vi "EXCOM-TCP-28.vi"(0 "connection ID":refnum<k5>, 5 "Error IN":errorcluster) -> (14 "CID Out":refnum<k5>, 15 "NORA":dbl format="%<%H:%M:%S%0u>t", 16 "NODEC":dbl format="%<%H:%M:%S%0u>t", 17 "DEC":dbl format="%.2f", 18 "HA":dbl format="%.2f", 19 "Error Out":errorcluster)   [LabVIEW 2011]
panel:
  out "Q String":string
  out "RA":dbl format="%<%H:%M:%S%0u>t"
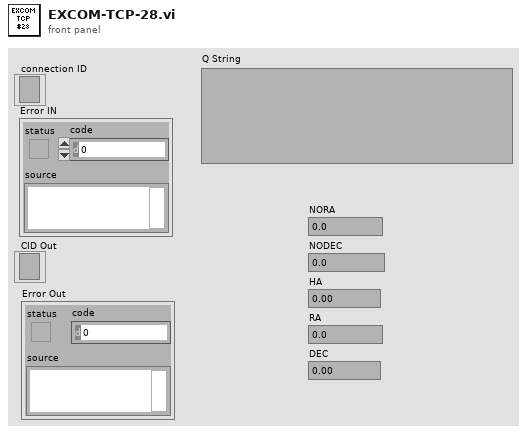
[diagram p1: front panel]
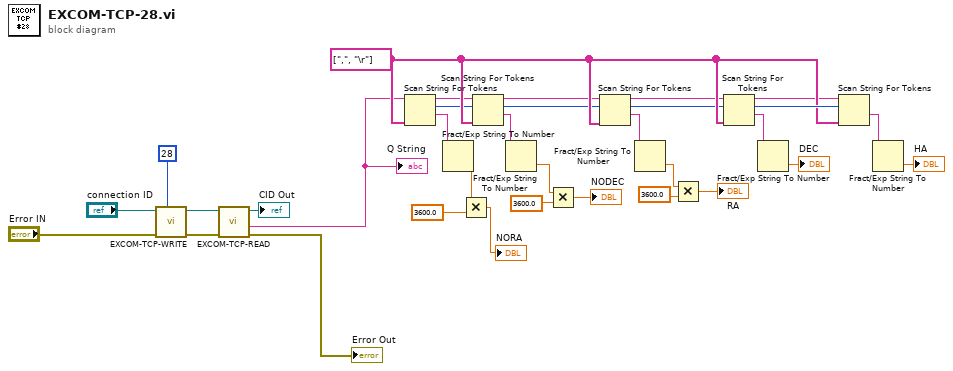
[diagram p0: block diagram]
diagram:
  w25 = string[] [",", "\r"] ("delimiters (\\s,\\t,\\r,\\n)")
  n1 = call "EXCOM-TCP-WRITE.vi"("Commande #"=28, "Error IN"="Error IN", "connection ID"="connection ID") -> ("Error OUT"=w31:errorcluster, "connection ID out"=w30:refnum<k5>)  [unwired: 4 in, 2 out]
  n2 = call "EXCOM-TCP-READ.vi"("Error In"=w31, "connection ID"=w30) -> ("Error Out"=→"Error Out":errorcluster, "Response"=w1:string, "CID Out"=→"CID Out":refnum<k5>)  [unwired: 5 in]
  "Q String" <- w1
  n3 = Scan String For Tokens(6:w25, 9:w1) -> (1:w8:string, 2:w7:i32, 3:w6:string)  [unwired: 4 in, 1 out]
  n4 = Fract/Exp String To Number(string=w8) -> (number=w9:dbl)  [unwired: 3 in, 1 out]
  n5 = Multiply(x=w9, y=3600.0) -> (x*y=→"NORA":dbl)
  n6 = Scan String For Tokens(6:w25, 8:w7, 9:w6) -> (1:w20:string, 2:w4:i32, 3:w5:string)  [unwired: 3 in, 1 out]
  n7 = Fract/Exp String To Number(string=w20) -> (number=w16:dbl)  [unwired: 3 in, 1 out]
  n8 = Multiply(x=w16, y=3600.0) -> (x*y=→"NODEC":dbl)
  n9 = Scan String For Tokens(6:w25, 8:w4, 9:w5) -> (1:w14:string, 2:w2:i32, 3:w3:string)  [unwired: 3 in, 1 out]
  n10 = Fract/Exp String To Number(string=w14) -> (number=w18:dbl)  [unwired: 3 in, 1 out]
  n11 = Multiply(x=w18, y=3600.0) -> (x*y=→"RA":dbl)
  n12 = Scan String For Tokens(6:w25, 8:w2, 9:w3) -> (1:w15:string, 2:w26:i32, 3:w24:string)  [unwired: 3 in, 1 out]
  n13 = Fract/Exp String To Number(string=w15) -> (number=→"DEC":dbl)  [unwired: 3 in, 1 out]
  n14 = Scan String For Tokens(6:w25, 8:w26, 9:w24) -> (1:w23:string)  [unwired: 3 in, 3 out]
  n15 = Fract/Exp String To Number(string=w23) -> (number=→"HA":dbl)  [unwired: 3 in, 1 out]
